vi "Dispose.vi"(8 "error in (no error)":errorcluster, 11 "RoomWithBomb":refnum<class "RoomWithBomb.lvclass">) -> (0 "error out":errorcluster)   [LabVIEW 2020, in "RoomWithBomb.lvclass"]
uses:
  RoomWithBomb.lvclass
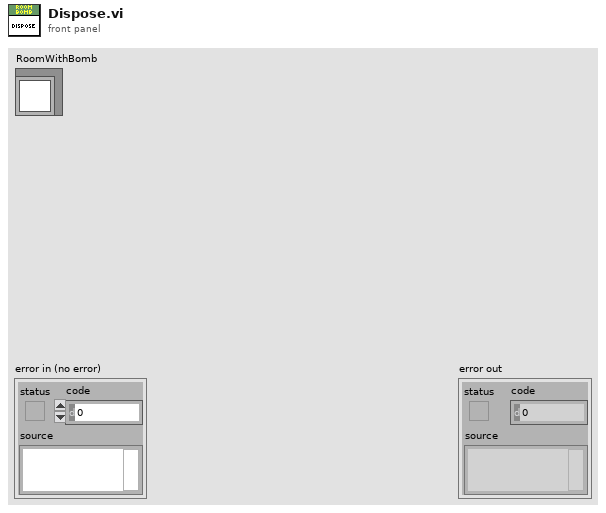
[diagram p1: front panel]
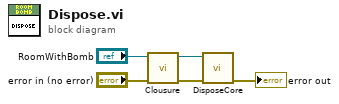
[diagram p0: block diagram]
diagram:
  n1 = call-dynamic "Clousure.vi"("error in (no error)"="error in (no error)", "RoomWithBomb"="RoomWithBomb") -> ("error out"=w2:errorcluster, "RoomWithBomb"=w3:refnum<class "RoomWithBomb.lvclass">)  [unwired: 8 in]
  n2 = call-dynamic "DisposeCore.vi"("error in (no error)"=w2, "RoomWithBomb"=w3) -> ("error out"=→"error out":errorcluster)  [unwired: 8 in, 1 out]
